vi "独立测试.vi"() -> ()   [LabVIEW 2017]
uses:
  HslCommunication.dll
panel:
  out "标签打印启动信号 8":bool
  out "标签打印启动信号 7":bool
  out "标签打印启动信号 6":bool
  out "标签打印启动信号 5":bool
  out "标签打印启动信号 4":bool
  out "标签打印启动信号 3":bool
  out "标签打印启动信号 2":bool
  out "IsSuccess":bool
  out "Content":u8[](array[numeric])
  in  "停止":bool
  out "标签打印启动信号":bool
  out "7":bool
  out "6":bool
  out "5":bool
  out "4":bool
  out "3":bool
  out "2":bool
  out "1":bool
  out "字符识别启动信号":bool
  out "通讯状态":bool
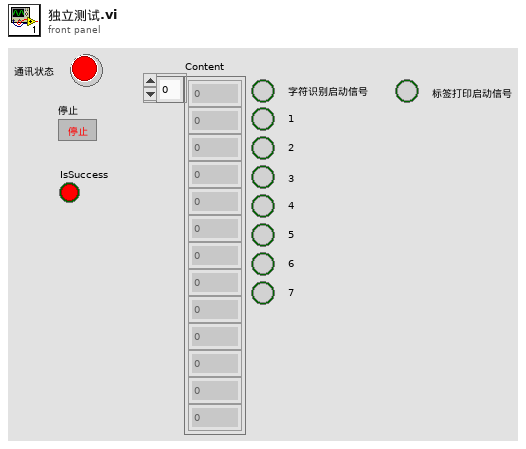
[diagram p1: front panel]
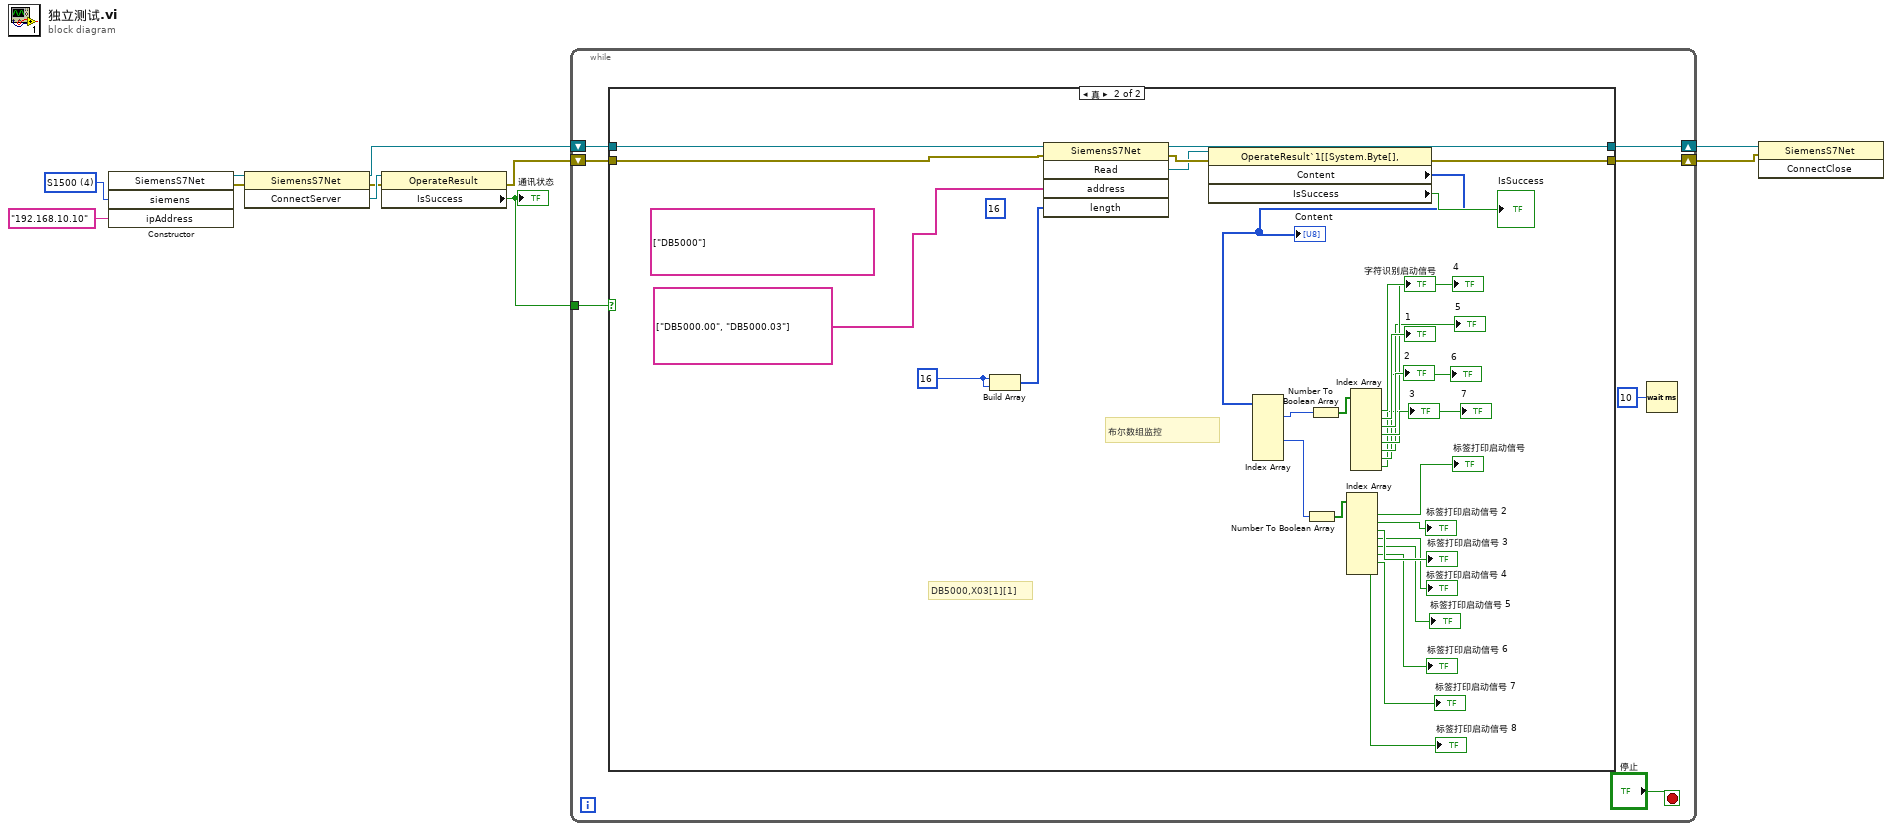
[diagram p0: block diagram]
diagram:
  w10 = 4 items=["S1200"=1, "S300"=2, "S400"=3, "S1500"=4, "S200Smart"=5] ("siemens")
  n1 = constructor class="SiemensS7Net"("siemens"=w10, "ipAddress"="192.168.10.10") -> (reference out=w8:refnum<k24>, error out=w7:errorcluster)  [unwired: 3 in, 3 out]
  n2 = invoke class="SiemensS7Net" method="ConnectServer"(reference=w8, error in=w7) -> (reference out=w3:refnum<k24>, error out=w6:errorcluster, "ConnectServer"=w11:refnum<k24>)  [unwired: 1 in]
  n3 = property class="OperateResult"(reference=w11, error in=w6) -> (error out=w4:errorcluster, "IsSuccess"=w5:bool)  [unwired: 1 out]
  "通讯状态" <- w5
  n4 = while {
    tunnel: w5 -> [w18]
    shift-right: [w15] -> w2
    shift-left: w3 -> [w17]
    shift-right: [w14] -> w1
    shift-left: w4 -> [w16]
    stop <- "停止" stop-if-true
    n5 = case shown="真" w18 {
      tunnel: w17 -> [w20 w51]
      tunnel: w16 -> [w19 w50]
      tunnel: [w20 w48] -> w15
      tunnel: [w19 w47] -> w14
      frame False {
      }
      frame True {
        (unwired) u16 16 ("length")
        (unwired) string[] ["DB5000"]
        w29 = u16 16
        # "布尔数组监控"
        # "DB5000,X03[1][1]"
        n6 = Build Array(w29, w29) -> (w44:u16[])
        n7 = invoke class="SiemensS7Net" method="Read"(reference=w51, error in=w50, "address"=string[] ["DB5000.00", "DB5000.03"], "length"=w44) -> (reference out=w48:refnum<k24>, error out=w49:errorcluster, "Read"=w46:refnum<k24>)  [unwired: 1 in, 2 out]
        n8 = property class="OperateResult`1[[System.Byte[],"(reference=w46, error in=w49) -> (error out=w47:errorcluster, "Content"=w32:u8[], "IsSuccess"=→"IsSuccess":bool)  [unwired: 1 out]
        "Content" <- w32
        n9 = Index Array(array=w32) -> (element #1=w42:u8, element #4=w28:u8)  [unwired: 6 in, 4 out]
        n10 = Number To Boolean Array(number=w28) -> (Boolean array=w31:bool[])
        n11 = Number To Boolean Array(number=w42) -> (Boolean array=w41:bool[])
        n12 = Index Array(array=w31) -> (element #1=→"标签打印启动信号":bool, element #2=→"标签打印启动信号 2":bool, element #3=→"标签打印启动信号 3":bool, element #4=→"标签打印启动信号 4":bool, element #5=→"标签打印启动信号 5":bool, element #6=→"标签打印启动信号 6":bool, element #7=→"标签打印启动信号 7":bool, element #8=→"标签打印启动信号 8":bool)  [unwired: 8 in]
        n13 = Index Array(array=w41) -> (element #1=→"字符识别启动信号":bool, element #2=→"1":bool, element #3=→"2":bool, element #4=→"3":bool, element #5=→"4":bool, element #6=→"5":bool, element #7=→"6":bool, element #8=→"7":bool)  [unwired: 8 in]
      }
    }
    n14 = Wait (ms)(milliseconds to wait=u32 10 ("等待时间（毫秒）")) -> ()  [unwired: 1 out]
  }
  n15 = invoke class="SiemensS7Net" method="ConnectClose"(reference=w2, error in=w1) -> ()  [unwired: 1 in, 3 out]
